vi "Subvi AO LUT mon.vi"(1 "mon":refnum<k21>="Connector1/AO1", 2 "AO":refnum<k21>="Connector1/AO0", 7 "Enable trigger":bool, 9 "FIFO In":refnum<k21>="GALVO1") -> ()   [LabVIEW 2017]
uses:
  <vilib>/Platform/TimedLoop/XDataNode/timing_clust.ctl
  <vilib>/Platform/TimedLoop/XDataNode/nitl_modes.ctl
  <vilib>/Platform/TimedLoop/XDataNode/wakeup.ctl
  <vilib>/rvi/Emulation/niFpgaSctlEmulationGetInTimedLoop.vi
  <vilib>/rvi/Emulation/niFpgaEmulationReportErrorSimple.vi
  <vilib>/rvi/Emulation/niFpgaGetClockAttributes.vi
  <vilib>/rvi/Emulation/niFpgaCriticalErrorInLSC.vi
  GV frameclock.vi
  GV trigger delay.vi
  GV frame counter.vi
  <vilib>/rvi/DataTransferAndStorage/Container/Common/niFpgaContainerExecOnDevCompGetState.vi
  <vilib>/rvi/Emulation/niFpgaEmulationIsFPGAContextNoSignature.vi
  <vilib>/rvi/DataTransferAndStorage/Container/Common/niFpgaContainerGetUniqueNameForEmu.vi
  <vilib>/rvi/Emulation/niFpgaProcessEmulError.vi
  <vilib>/rvi/errors/nirviReportUnexpectedCaseInternalError (U32).vi
  <vilib>/rvi/Memory/Memory_Emulation/niFpgaMemoryEmulationCacheClearOnFirstRun.vi
  <vilib>/rvi/Memory/Memory_Emulation/nirvimemoryEmulationManagerCache_MakeExclusive.vi
  <vilib>/rvi/Memory/Memory_Emulation/niFpgaMemoryEmulationValidateCache.vi
  <vilib>/rvi/Memory/Memory_Emulation/nirvimemoryEmulationManagerCache_InsertValue.vi
  <vilib>/Utility/error.llb/Clear Errors.vi
  <vilib>/rvi/Memory/Memory_Emulation/nirvimemoryEmulationManagerCache_ReleaseExclusive.vi
  <vilib>/rvi/Memory/Memory_Emulation/nirvimemoryEmulationManagerCache_GetValue.vi
  <vilib>/rvi/Memory/Memory_Emulation/nirvimemoryEmulationManagerCache_SetValue.vi
  <vilib>/rvi/Emulation/niFpgaSctlEmulationResourceMgr.vi
  <vilib>/rvi/eio/common/nirviEmuTemplateMethod_errors.vi
  <vilib>/Platform/TimedLoop/XDataNode/XDataNode.xnode
  <vilib>/rvi/DataTransferAndStorage/Container/XNode/niFpgaContainer.xnode
  <vilib>/rvi/Memory/Memory_Emulation/niFpgaMemoryEmulationRefIn.vi
  <vilib>/eio/EIONode/EIONode.xnode
  <vilib>/Platform/TimedLoop/XDataNode/XDNodeRunTimeDep.lvlib
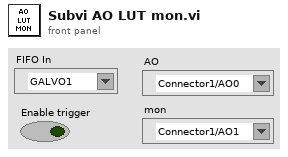
[diagram p1: front panel]
types:
  T1 = typedef "XDNodeRunTimeDep.lvlib/timing_clust.ctl" = cluster{"Expected End [f-1]":u64, "Actual End [f-1]":u64, "Finished Late? [f-1]":bool, "Expected End [i-1]":u64, "Actual End [i-1]":u64, "Finished Late? [i-1]":bool, "Expected Start [i]":u64, "Actual Start [i]":u64, "Expected Start [f]":u64, "Actual Start [f]":u64, "Source Name":string, "Structure Name":string, "Period":i64, "Deadline":i64, "Offset":i64, "Start":i64, "Priority":i32, "Timeout":i32, "Mode":T2, "Wakeup Reason":T3, "Error":errorcluster, "Source Type":string, "Secondary Source Type":string, "Global End Time":u64, "Global Start Time":u64, "Frame Duration":u64, "Iteration Duration":u64, "Assigned CPU":i32, "I/O Scan Engine Mode":u32}
  T2 = typedef "XDNodeRunTimeDep.lvlib/nitl_modes.ctl" = enum32{"No Change", "Process missed periods, maintain original phase", "Discard missed periods, maintain original phase", "Process missed periods, ignore original phase", "Discard missed periods, ignore original phase"}
  T3 = typedef "XDNodeRunTimeDep.lvlib/wakeup.ctl" = enum32{"Normal", "Aborted", "Asynchronous wakeup", "Timing source error", "Timed loop error", "Timeout"}
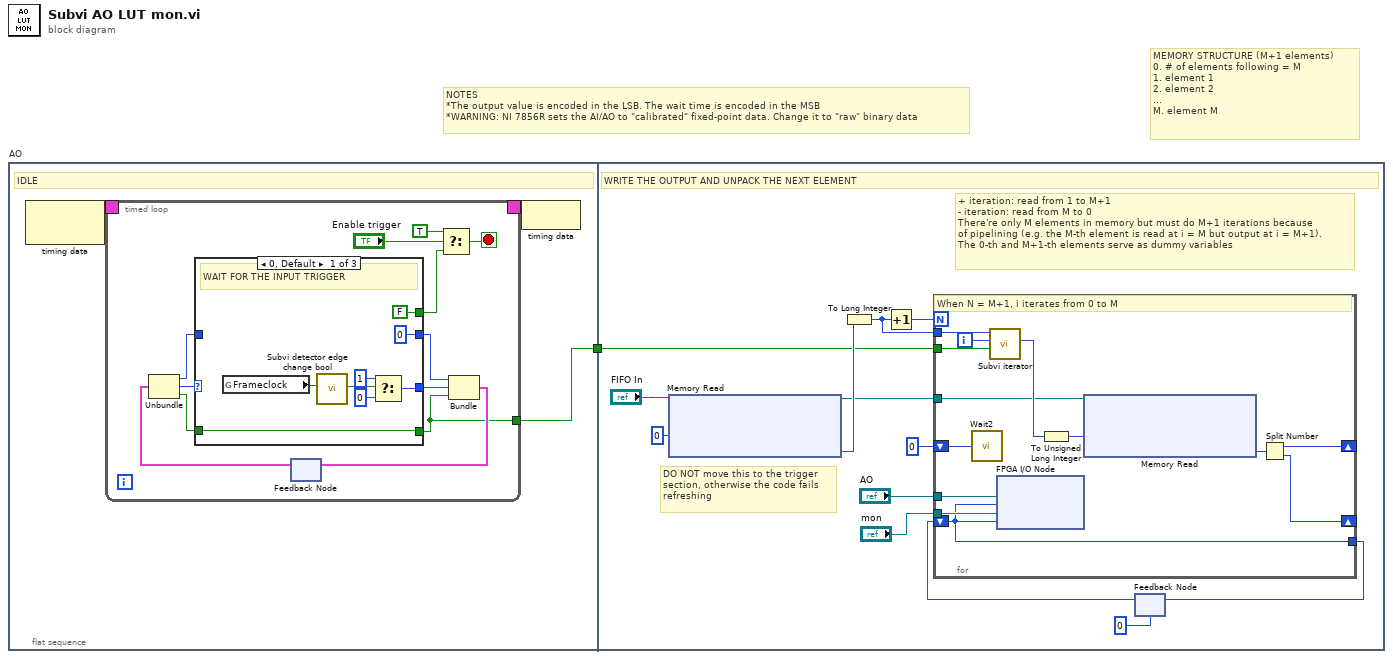
[diagram p0: block diagram]
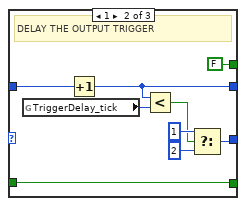
[diagram p2: hidden frame]
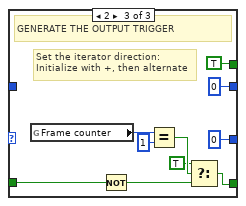
[diagram p3: hidden frame]
diagram:
  # "MEMORY STRUCTURE (M+1 elements)\n0. # of elements following = M\n1. element 1\n2. element 2\n...\nM. element M"
  # "NOTES\n*The output value is encoded in the LSB. The wait time is encoded in the MSB\n*WARNING: NI 7856R sets the AI/AO to \"calibrated\" fixed-point data. Change it to \"raw\" binary data"
  n1 = flat-sequence "AO" {
    tunnel: [w4] -> w1
    tunnel: w1 -> [w53]
    frame #0 {
      # "IDLE"
      n2 = node-c288() -> (w3:T1)  [unwired: 1 in]
      n3 = timed-loop {
        timing: w3 -> [_]
        timing-out: [_] -> w2
        tunnel: [w6] -> w4
        stop <- w16 stop-if-true
        n4 = feedback #1() -> (w11:cluster{u16, "f":u8, bool})  [unwired: 1 in]
        n5 = Unbundle(w11) -> (w10:u16, "f"=w8:u8, w7:bool)
        n6 = case shown="0, Default" w8 {
          tunnel: [u16 0 w31 u16 0] -> w14
          tunnel: [w24 w27 u8 0 ("f")] -> w9
          tunnel: w10 -> [_ w32 _]
          tunnel: [FALSE FALSE TRUE] -> w13
          tunnel: [w19 w25 w34] -> w6
          tunnel: w7 -> [w19 w25 w36]
          frame 0, Default {
            # "WAIT FOR THE INPUT TRIGGER"
            n7 = global read "GV frameclock.vi" "Frameclock"() -> (w17:bool)
            n8 = call "Subvi detector edge change bool.vi"("Input"=w17) -> ("Output"=w18:bool)  [unwired: 8 in]
            n9 = Select(t=u8 1, s=w18, f=u8 0) -> (s? t:f=w24:u8)
          }
          frame 1 {
            # "DELAY THE OUTPUT TRIGGER"
            n10 = global read "GV trigger delay.vi" "TriggerDelay_tick"() -> (w33:u16)
            n11 = Increment(x=w32) -> (x+1=w31:u16)
            n12 = Less?(x=w31, y=w33) -> (x < y?=w29:bool)
            n13 = Select(t=u8 1, s=w29, f=u8 2) -> (s? t:f=w27:u8)
          }
          frame 2 {
            # "Set the iterator direction:\nInitialize with +, then alternate"
            # "GENERATE THE OUTPUT TRIGGER"
            n14 = global read "GV frame counter.vi" "Frame counter"() -> (w38:u8)
            n15 = Not(x=w36) -> (.not. x?=w35:bool)
            n16 = Equal?(x=w38, y=u8 1) -> (x = y?=w40:bool)
            n17 = Select(t=TRUE, s=w40, f=w35) -> (s? t:f=w34:bool)
          }
        }
        n18 = Select(t=TRUE, s="Enable trigger", f=w13) -> (s? t:f=w16:bool)
        n19 = Bundle(w14, "f"=w9, w6) -> (w12:cluster{u16, "f":u8, bool})  [unwired: 1 in]
        n20 = feedback-in #1(w12) -> ()
      }
      n21 = node-c288(w2) -> ()
    }
    frame #1 {
      # "+ iteration: read from 1 to M+1\n- iteration: read from M to 0\nThere're only M elements in memory but must do M+1 iterations because \nof pipelining (e.g. the M-th element is read at i = M but output at i = M+1).\nThe 0-th and M+1-th elements serve as dummy variables"
      # "DO NOT move this to the trigger\nsection, otherwise the code fails\nrefreshing"
      # "WRITE THE OUTPUT AND UNPACK THE NEXT ELEMENT"
      n22 = xnode ("Memory Read")("Address"=u32 0, "Memory In"="FIFO In") -> ("Data"=w59:u32, "Memory Out"=w58:refnum<k21>)
      n23 = To Long Integer(number=w59) -> (32bit integer=w51:i32)
      n24 = Increment(x=w51) -> (x+1=w52:i32)
      n25 = feedback #2(u16 0) -> (w49:u16)
      n26 = for {
        N: w52 -> [_]
        shift-right: [w71] -> _
        shift-left: u16 0 -> [w69]
        shift-right: [w70] -> _
        shift-left: w49 -> [w61]
        tunnel: [w61] -> w50
        tunnel: w51 -> [w66]
        tunnel: w58 -> [w65]
        tunnel: "AO" -> [w62]
        tunnel: w53 -> [w64]
        tunnel: "mon" -> [w63]
        i -> [w67]
        # "When N = M+1, i iterates from 0 to M"
        n27 = call "Wait2"("Count(Ticks)"=w69) -> ()  [unwired: 1 out]
        n28 = call "Subvi iterator.vi"("Set increase"=w64, "Iterator in"=w67, "Nmax"=w66) -> ("Iterator out"=w68:i32)  [unwired: 8 in]
        n29 = xnode ("FPGA I/O Node")("I/O Item"=w61, "FPGA I/O In"=w62, "I/O Item"=w61, "FPGA I/O In"=w63) -> ()  [unwired: 2 out]
        n30 = To Unsigned Long Integer(number=w68) -> (unsigned 32bit integer=w73:u32)
        n31 = xnode ("Memory Read")("Address"=w73, "Memory In"=w65) -> ("Data"=w72:u32)  [unwired: 1 out]
        n32 = Split Number(x=w72) -> (hi(x)=w71:u16, lo(x)=w70:u16)
      }
      n33 = feedback-in #2(w50) -> ()
    }
  }
